vi "Check parts acceptable.vi"(8 "error in (no error)":errorcluster, 9 "Baselayer IDs":string[](array[string]), 10 "DB out":string[][](array[string]), 11 "Database Entry in":refnum<class "Database Entry.lvclass">) -> (0 "error out":errorcluster, 1 "Thickness out":string[](array[string]), 3 "Database Entry out":refnum<class "Database Entry.lvclass">, 4 "Abort?":bool)   [LabVIEW 2021, in "Database Entry.lvclass"]
uses:
  Database Entry.lvclass
  Database Entry.lvclass/Database Entry.ctl
  Components/Stack/Stack.lvclass
panel:
  in  "Thickness column options to use for assembly":u16(ring) items=["thickness"]
  in  "Are these parts satisfactory?":bool
  in  "Abort":bool
  in  "Submit":bool
  in  "Proposed thickness for assembly dispense":string[](array[string])
  in  "Database out":i32[](listbox)
  # "Modify thickness values manually, if needed"
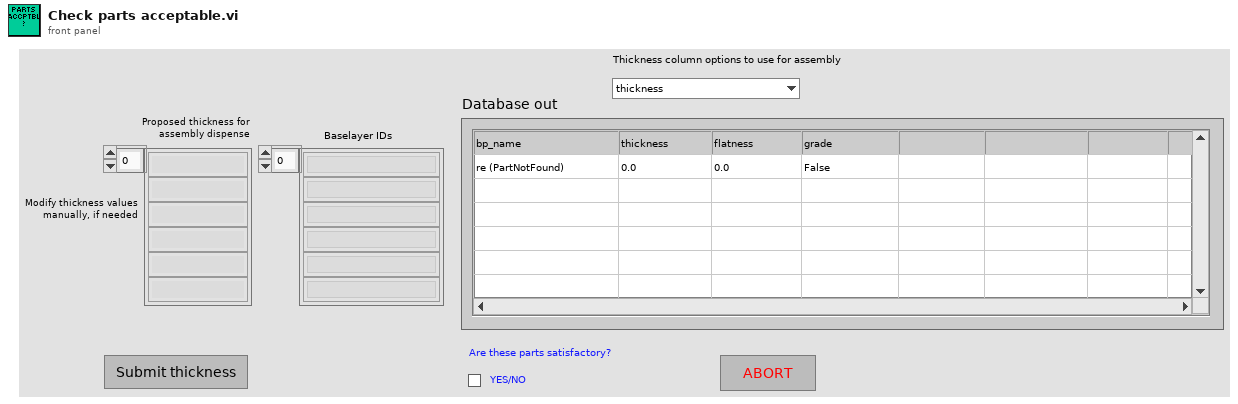
[diagram p1: front panel]
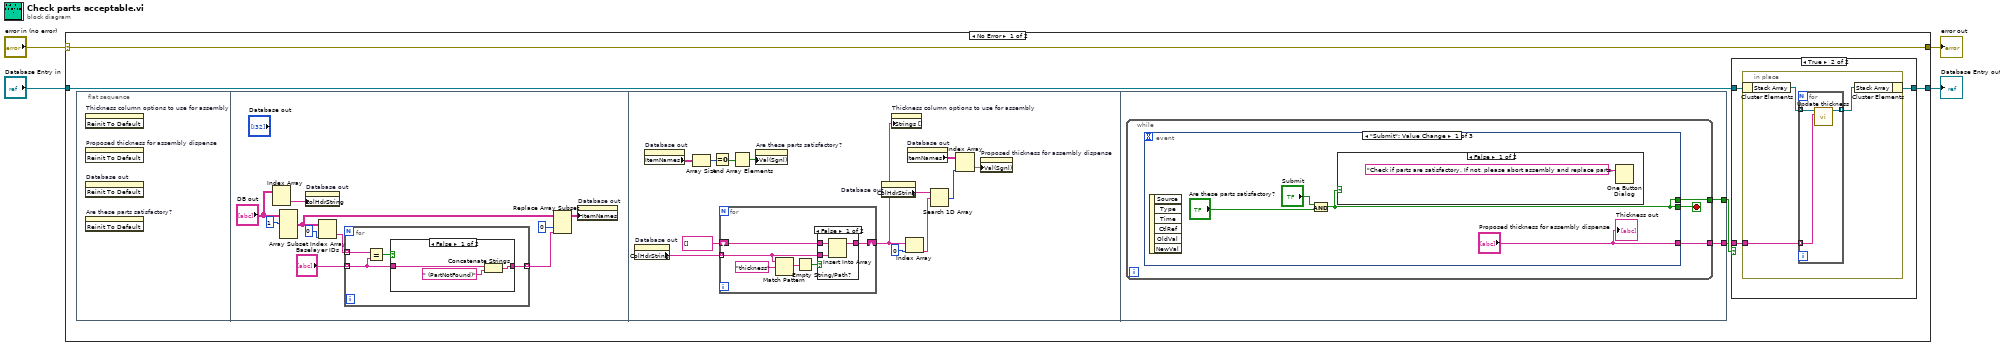
[diagram p0: block diagram]
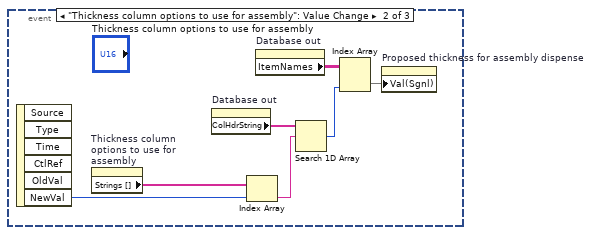
[diagram p5: hidden frame]
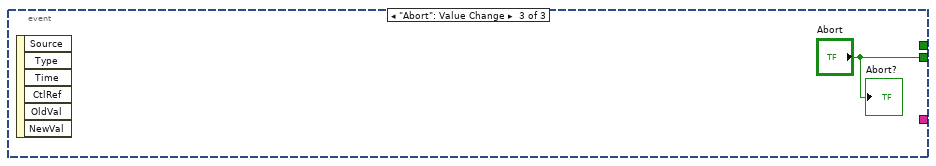
[diagram p6: hidden frame]
diagram:
  n1 = case shown="No Error" "error in (no error)" {
    selector: "error in (no error)" -> [w9 w80]
    tunnel: [w9 w80] -> w3
    tunnel: [w7 w79] -> w1
    tunnel: "Database Entry in" -> [w6 w79]
    frame No Error {
      n2 = flat-sequence {
        tunnel: [w52] -> w8
        tunnel: [w51] -> w5
        frame #0 {
          n3 = invoke on="Thickness column options to use for assembly" class="Ring (strict)" method="Reinit To Default"() -> ()  [unwired: 3 in, 3 out]
          n4 = invoke on="Proposed thickness for assembly dispense" class="Arr (strict)" method="Reinit To Default"() -> ()  [unwired: 3 in, 3 out]
          n5 = invoke on="Database out" class="MCListbox (strict)" method="Reinit To Default"() -> ()  [unwired: 3 in, 3 out]
          n6 = invoke on="Are these parts satisfactory?" class="Bool (strict)" method="Reinit To Default"() -> ()  [unwired: 3 in, 3 out]
        }
        frame #1 {
          n7 = Index Array(array="DB out") -> (element=w11:string[])  [unwired: 2 in]
          n8 = Array Subset(array="DB out", index (row)=1 ("index")) -> (w16:string[][])  [unwired: 3 in]
          n9 = property on="Database out" class="MCListbox (strict)"("ColHdrString"=w11) -> ()  [unwired: 2 in, 2 out]
          n10 = Index Array(array=w16, index (col)=0 ("disabled index (col)")) -> (element=w17:string[])  [unwired: 1 in]
          n11 = for {
            tunnel: w17 -> [w22] mode=indexing
            tunnel: "Baselayer IDs" -> [w20] mode=indexing
            tunnel: [w21] -> w14 mode=indexing
            n12 = Equal?(x=w22, y=w20) -> (x = y?=w23:bool)
            n13 = case shown="False" w23 {
              tunnel: w20 -> [w26 w27]
              tunnel: [w24 w27] -> w21
              frame False {
                n14 = Concatenate Strings(w26, " (PartNotFound)" ("string")) -> (w24:string)
              }
              frame True {
              }
            }
          }
          n15 = Replace Array Subset(array=w16, new element=w14, index (col)=0 ("disabled index (col)")) -> (w10:string[][])  [unwired: 1 in]
          n16 = property on="Database out" class="MCListbox (strict)"("ItemNames"=w10) -> ()  [unwired: 2 in, 2 out]
        }
        frame #2 {
          n17 = property on="Database out" class="MCListbox (strict)"() -> ("ColHdrString"=w36:string[])  [unwired: 2 in, 2 out]
          n18 = property on="Database out" class="MCListbox (strict)"() -> ("ItemNames"=w28:string[][])  [unwired: 2 in, 2 out]
          n19 = Array Size(array=w28) -> (size(s)=w29:i32[])
          n20 = Equal To 0?(x=w29) -> (x = 0?=w30:bool[])
          n21 = for {
            tunnel: w36 -> [w43] mode=indexing
            shift-right: [w42] -> w37
            shift-left: string[] [] -> [w41]
            n22 = Match Pattern(string=w43, regular expression="thickness") -> (match substring=w45:string)  [unwired: 1 in, 3 out]
            n23 = Empty String/Path?(string/path=w45) -> (empty?=w44:bool)
            n24 = case shown="False" w44 {
              tunnel: [w47 w50] -> w42
              tunnel: w43 -> [w48 _]
              tunnel: w41 -> [w49 w50]
              frame False {
                n25 = Insert Into Array(array=w49, new element=w48) -> (w47:string[])  [unwired: 1 in]
              }
              frame True {
              }
            }
          }
          n26 = And Array Elements(Boolean array=w30) -> (logical AND=w31:bool)
          n27 = property on="Are these parts satisfactory?" class="Bool (strict)"("Val(Sgnl)"=w31) -> ()  [unwired: 2 in, 2 out]
          n28 = property on="Database out" class="MCListbox (strict)"() -> ("ColHdrString"=w38:string[])  [unwired: 2 in, 2 out]
          n29 = property on="Thickness column options to use for assembly" class="Ring (strict)"("Strings []"=w37) -> ()  [unwired: 2 in, 2 out]
          n30 = Index Array(array=w37, index=0) -> (element=w39:string)
          n31 = property on="Database out" class="MCListbox (strict)"() -> ("ItemNames"=w40:string[][])  [unwired: 2 in, 2 out]
          n32 = Search 1D Array(1D array=w38, element=w39) -> (index of element=w32:i32)  [unwired: 1 in]
          n33 = Index Array(array=w40, index (col)=w32) -> (element=w33:string[])  [unwired: 1 in]
          n34 = property on="Proposed thickness for assembly dispense" class="Arr (strict)"("Val(Sgnl)"=w33) -> ()  [unwired: 2 in, 2 out]
        }
        frame #3 {
          n35 = while {
            tunnel: [w53] -> w52
            tunnel: [w55] -> w51
            stop <- w54 stop-if-true
            n36 = event shown="[0] \"Submit\": Value Change" {
              selector: _ -> [_ _ _]
              dyn-events: _ -> [_ _ _]
              timeout: _ -> [_ _ _]
              tunnel: [w56 _ "Abort"] -> w54
              tunnel: ["Proposed thickness for assembly dispense" _ _] -> w55
              tunnel: [w56 _ _] -> w53
              event "Submit": Value Change {
                n37 = event-data() -> ()  [unwired: 1 in, 6 out]
                n38 = And(x="Submit", y="Are these parts satisfactory?") -> (x .and. y?=w56:bool)
                n39 = case shown="False" w56 {
                  frame False {
                    n40 = One Button Dialog(message="Check if parts are satisfactory. If not, please abort assembly and replace parts. ") -> ()  [unwired: 1 in, 1 out]
                  }
                  frame True {
                  }
                }
                "Thickness out" <- "Proposed thickness for assembly dispense"
              }
              event "Thickness column options to use for assembly": Value Change {
                n41 = event-data() -> ("NewVal"=w66:u16)  [unwired: 1 in, 5 out]
                n42 = property on="Thickness column options to use for assembly" class="Ring (strict)"() -> ("Strings []"=w67:string[])  [unwired: 2 in, 2 out]
                n43 = property on="Database out" class="MCListbox (strict)"() -> ("ColHdrString"=w62:string[])  [unwired: 2 in, 2 out]
                n44 = Index Array(array=w67, index=w66) -> (element=w65:string)
                n45 = property on="Database out" class="MCListbox (strict)"() -> ("ItemNames"=w64:string[][])  [unwired: 2 in, 2 out]
                n46 = Search 1D Array(1D array=w62, element=w65) -> (index of element=w61:i32)  [unwired: 1 in]
                n47 = Index Array(array=w64, index (col)=w61) -> (element=w63:string[])  [unwired: 1 in]
                n48 = property on="Proposed thickness for assembly dispense" class="Arr (strict)"("Val(Sgnl)"=w63) -> ()  [unwired: 2 in, 2 out]
              }
              event "Abort": Value Change {
                n49 = event-data() -> ()  [unwired: 1 in, 6 out]
                "Abort?" <- "Abort"
              }
            }
          }
        }
      }
      n50 = case shown="True" w8 {
        tunnel: [w69 w72] -> w7
        tunnel: w6 -> [w69 w71]
        tunnel: w5 -> [_ w70]
        frame False {
        }
        frame True {
          n51 = in-place {
            in-place-border: w70 -> [w73]
            n52 = in-place-cluster #1(w71) -> ("Stack Array"=w75:refnum<class "Stack.lvclass">[])
            n53 = for {
              tunnel: w75 -> [w78] mode=indexing
              tunnel: [w77] -> w74 mode=indexing
              tunnel: w73 -> [w76] mode=indexing
              n54 = call "Update thickness.vi"("Thickness"=w76, "Stack in"=w78) -> ("Stack out"=w77:refnum<class "Stack.lvclass">)  [unwired: 8 in, 1 out]
            }
            n55 = in-place-cluster #1("Stack Array"=w74) -> (w72:refnum<class "Database Entry.lvclass">)
          }
        }
      }
    }
    frame Error {
    }
  }
  "error out" <- w3
  "Database Entry out" <- w1
